vi "G#Object_ExternalCreateProcessDelegate.vi"(0 "delegate event out":refnum<user-event>, 1 "event queue":refnum<queue>, 5 "error in (no error)":errorcluster) -> (19 "error out":errorcluster)   [LabVIEW 2017, in "G#Object.lvclass"]
doc: "This is a delegate process that creates the object specified by the events."
uses:
  G#Object.lvclass
  utils/G#Object_Event.ctl
  utils/G#Object_EventType.ctl
  utils/G#Object_ObjectInfoType.ctl
  utils/G#Object_CreateMethod.ctl
  <vilib>/Utility/error.llb/Error Cluster From Error Code.vi
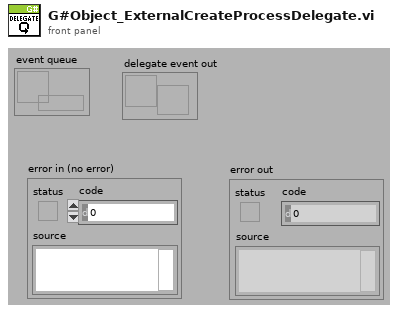
[diagram p1: front panel]
types:
  T1 = typedef "G#Object.lvclass/G#Object_EventType.ctl" = enum16{"Created new", "Looked up existing", "Deleted", "Forced delete", "Not deleted", "Garbage collected", "Cleared", "User", "Error", "External create object", "External create class attributes", "Created class attributes", "Run constructor", "Run constructor done", "Run open method", "Run open method done"}
  T2 = typedef "G#Object.lvclass/G#Object_ObjectInfoType.ctl" = cluster{"ObjectName":string, "ObjectID":u32, "Users":i32, "Counter":bool, "AttributeRefs":u32[], "FullClassName":string, "ClassName":string, "CreateMethod":T3, "GenericDestructorExists":bool, "Owner":string}
  T3 = typedef "G#Object.lvclass/G#Object_CreateMethod.ctl" = enum16{"Create", "Create or look up existing", "Look up existing"}
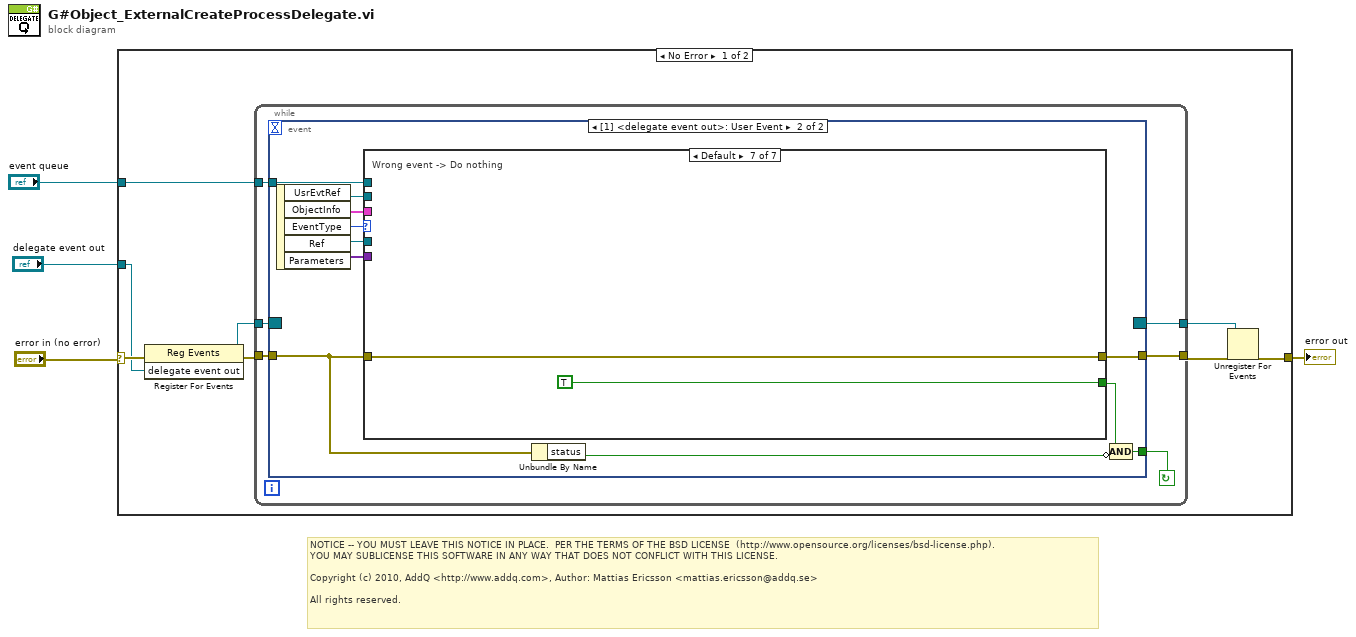
[diagram p0: block diagram]
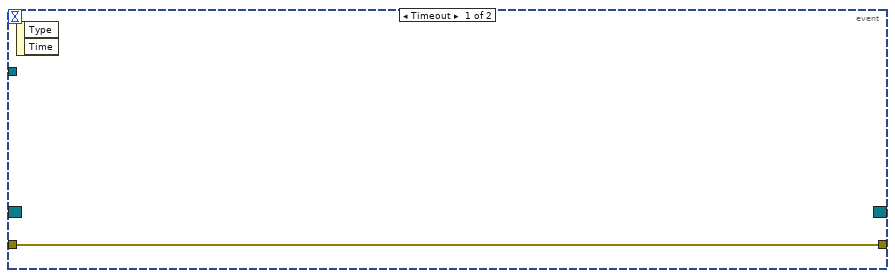
[diagram p2: hidden frame]
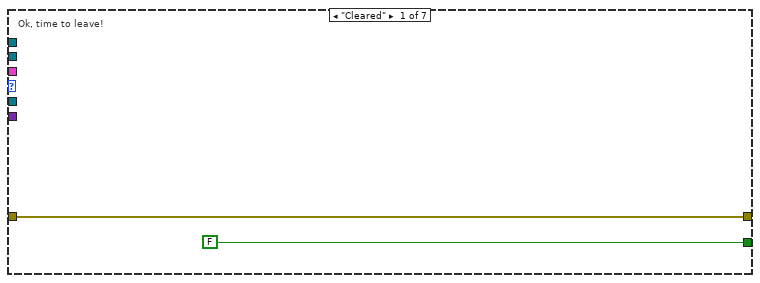
[diagram p3: hidden frame]
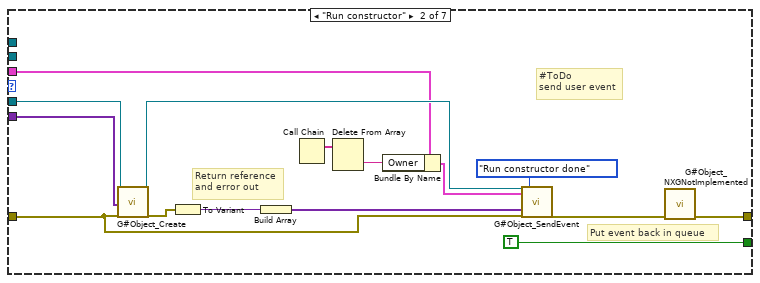
[diagram p4: hidden frame]
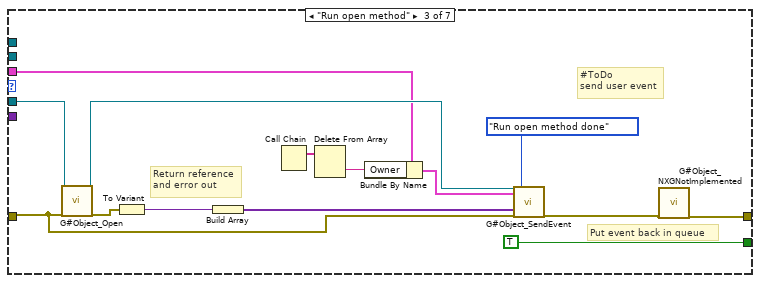
[diagram p5: hidden frame]
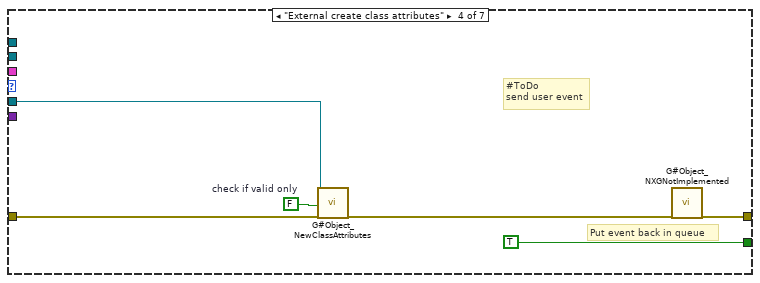
[diagram p6: hidden frame]
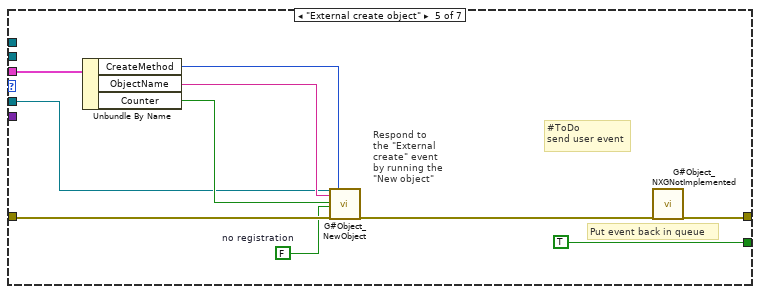
[diagram p7: hidden frame]
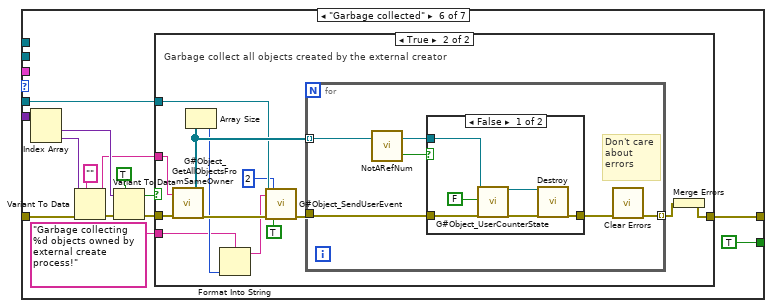
[diagram p8: hidden frame]
diagram:
  # "NOTICE -- YOU MUST LEAVE THIS NOTICE IN PLACE.  PER THE TERMS OF THE BSD LICENSE  (http://www.opensource.org/licenses/bsd-license.php).\nYOU MAY SUBLICENSE THIS SOFTWARE IN ANY WAY THAT DOES NOT CONFLICT WITH THIS LICENSE.\n\nCopyright (c) 2010, AddQ <http://www.addq.com>, Author: Mattias Ericsson <mattias.ericsson@addq.se>\n\nAll rights reserved."
  n1 = case shown="No Error" "error in (no error)" {
    selector: "error in (no error)" -> [w9 w121]
    tunnel: [w11 w121] -> w4
    tunnel: "event queue" -> [w12 _]
    tunnel: "delegate event out" -> [w8 _]
    frame No Error {
      n2 = register-events(error in=w9, w8) -> (reference out=w6:refnum<event-registration>, error out=w7:errorcluster)  [unwired: 1 in]
      n3 = while {
        tunnel: w7 -> [w18]
        tunnel: [w17] -> w10
        tunnel: w12 -> [w15]
        tunnel: w6 -> [w14]
        tunnel: [w13] -> w5
        stop <- w16 continue-if-true
        n4 = event shown="[1] <delegate event out>: User Event" {
          selector: w14 -> [_ _]
          dyn-events: [_ _] -> w13
          timeout: _ -> [_ _]
          tunnel: w18 -> [w19 w28]
          tunnel: [w19 w30] -> w17
          tunnel: [_ w25] -> w16
          tunnel: w15 -> [_ w22]
          event Timeout {
            n5 = event-data() -> ()  [unwired: 1 in, 2 out]
          }
          event User Event {
            n6 = event-data() -> ("UsrEvtRef"=w21:refnum<user-event>, "ObjectInfo"=w23:T2, "EventType"=w29:T1, "Ref"=w20:refnum<class "G#Object.lvclass">, "Parameters"=w24:variant[])  [unwired: 1 in]
            n7 = case shown="Default" w29 {
              tunnel: w28 -> [w32 w40 w54 w65 w73 w88 w119]
              tunnel: [w32 w33 w48 w62 w68 w90 w119] -> w30
              tunnel: [FALSE TRUE TRUE TRUE TRUE TRUE TRUE] -> w26
              tunnel: w24 -> [_ w35 _ _ _ w91 _]
              tunnel: w23 -> [_ w39 w51 _ w74 _ _]
              tunnel: w22 -> [_ _ _ _ _ _ _]
              tunnel: w21 -> [_ _ _ _ _ _ _]
              tunnel: w20 -> [_ w42 w56 w66 w71 w79 _]
              frame "Cleared" {
                # "Ok, time to leave!"
              }
              frame "Run constructor" {
                # "#ToDo\nsend user event"
                # "Put event back in queue"
                # "Return reference\nand error out"
                n8 = call-dynamic "G#Object_Create.vi"("reference in"=w42, "control values"=w35, "error in (no error)"=w40) -> ("reference out"=w41:refnum<class "G#Object.lvclass">, "error out"=w46:errorcluster)  [unwired: 15 in]
                n9 = To Variant(anything=w46) -> (Variant=w45:variant)
                n10 = Build Array(w45) -> (w43:variant[])
                n11 = Call Chain() -> (call chain=w37:string[])
                n12 = Delete From Array(array=w37) -> (deleted portion=w36:string)  [unwired: 2 in, 1 out]
                n13 = Bundle By Name(cluster=w39, "Owner"=w36) -> (w38:T2)
                n14 = call "G#Object_SendEvent.vi"("reference in"=w41, "object info extended"=w38, "parameters"=w43, "error in (no error)"=w40, "G# event type"=G#Object_EventType."Run constructor done") -> ("error out"=w34:errorcluster)  [unwired: 14 in]
                n15 = call "G#Object_NXGNotImplemented.vi"("error in"=w34) -> ("error out"=w33:errorcluster)  [unwired: 18 in]
              }
              frame "Run open method" {
                # "#ToDo\nsend user event"
                # "Put event back in queue"
                # "Return reference\nand error out"
                n16 = call-dynamic "G#Object_Open.vi"("reference in"=w56, "error in (no error)"=w54) -> ("reference out"=w55:refnum<class "G#Object.lvclass">, "error out"=w60:errorcluster)  [unwired: 16 in]
                n17 = To Variant(anything=w60) -> (Variant=w59:variant)
                n18 = Build Array(w59) -> (w57:variant[])
                n19 = Call Chain() -> (call chain=w53:string[])
                n20 = Delete From Array(array=w53) -> (deleted portion=w52:string)  [unwired: 2 in, 1 out]
                n21 = Bundle By Name(cluster=w51, "Owner"=w52) -> (w50:T2)
                n22 = call "G#Object_SendEvent.vi"("reference in"=w55, "object info extended"=w50, "parameters"=w57, "error in (no error)"=w54, "G# event type"=G#Object_EventType."Run open method done") -> ("error out"=w49:errorcluster)  [unwired: 14 in]
                n23 = call "G#Object_NXGNotImplemented.vi"("error in"=w49) -> ("error out"=w48:errorcluster)  [unwired: 18 in]
              }
              frame "External create class attributes" {
                w64 = FALSE  # check if valid only
                # "#ToDo\nsend user event"
                # "Put event back in queue"
                n24 = call "G#Object_NewClassAttributes.vi"("reference in"=w66, "check if valid only (F)"=w64, "error in (no error)"=w65) -> ("error out"=w63:errorcluster)  [unwired: 12 in, 4 out]
                n25 = call "G#Object_NXGNotImplemented.vi"("error in"=w63) -> ("error out"=w62:errorcluster)  [unwired: 18 in]
              }
              frame "External create object" {
                w70 = FALSE  # no registration
                # "#ToDo\nsend user event"
                # "Put event back in queue"
                # "Respond to\nthe \"External\ncreate\" event\nby running the\n\"New object\""
                n26 = Unbundle By Name(w74) -> ("CreateMethod"=w77:T3, "ObjectName"=w76:string, "Counter"=w75:bool)
                n27 = call "G#Object_NewObject.vi"("reference in"=w71, "object name (\"\")"=w76, "user counter (T)"=w75, "no registration (F)"=w70, "error in (no error)"=w73, "create method"=w77) -> ("error out"=w69:errorcluster)  [unwired: 11 in, 2 out]
                n28 = call "G#Object_NXGNotImplemented.vi"("error in"=w69) -> ("error out"=w68:errorcluster)  [unwired: 18 in]
              }
              frame "Garbage collected" {
                n29 = Index Array(array=w91) -> (element #1=w84:variant, element #2=w85:variant)  [unwired: 2 in]
                n30 = Variant To Data(error in=w88, type="", Variant=w85) -> (data=w80:string, error out=w87:errorcluster)
                n31 = Variant To Data(error in=w87, type=TRUE, Variant=w84) -> (data=w81:bool, error out=w86:errorcluster)
                n32 = case shown="True" w81 {
                  tunnel: [w92 w105] -> w90
                  tunnel: w86 -> [w92 w103]
                  tunnel: w80 -> [_ w102]
                  tunnel: w79 -> [_ w98]
                  tunnel: "Garbage collecting %d objects owned by external create process!" -> [_ w95]
                  frame False {
                  }
                  frame True {
                    # "Garbage collect all objects created by the external creator"
                    n33 = call "G#Object_GetAllObjectsFromSameOwner.vi"("full class name (\"\")"=w102, "error in (no error)"=w103) -> ("all refs"=w101:refnum<class "G#Object.lvclass">[], "error out"=w100:errorcluster)  [unwired: 14 in, 2 out]
                    n34 = Array Size(array=w101) -> (size(s)=w97:i32)
                    n35 = Format Into String(format string=w95, w97) -> (resulting string=w96:string)  [unwired: 2 in, 1 out]
                    n36 = call "G#Object_SendUserEvent.vi"("refererence in"=w98, "text"=w96, "error in (no error)"=w100, "call depth (1)"=2 ("call depth"), "send to Desktop Trace Execution? (F)"=TRUE ("send to Desktop Trace Execution")) -> ("error out"=w99:errorcluster)  [unwired: 13 in, 1 out]
                    n37 = for {
                      tunnel: w99 -> [w106]
                      tunnel: [w110] -> w104 mode=indexing
                      tunnel: w101 -> [w109] mode=indexing
                      # "Don't care\nabout\nerrors"
                      n38 = call-dynamic "NotARefNum.vi"("reference in"=w109) -> ("not a refnum?"=w108:bool, "reference out"=w107:refnum<class "G#Object.lvclass">)  [unwired: 1 in]
                      n39 = case shown="False" w108 {
                        tunnel: [w117 w118] -> w111
                        tunnel: w106 -> [w116 w118]
                        tunnel: w107 -> [w114 _]
                        frame False {
                          n40 = call "G#Object_UserCounterState.vi"("reference in"=w114, "user counter (F)"=FALSE, "error in (no error)"=w116) -> ("reference out"=w112:refnum<class "G#Object.lvclass">, "error out"=w115:errorcluster)  [unwired: 15 in]
                          n41 = call-dynamic "Destroy.vi"("reference in"=w112, "error in (no error)"=w115) -> ("error out"=w117:errorcluster)  [unwired: 16 in, 1 out]
                        }
                        frame True {
                        }
                      }
                      n42 = call <vilib>:"Clear Errors.vi"("error in (no error)"=w111) -> ("error out"=w110:errorcluster)  [unwired: 5 in, 1 out]
                    }
                    n43 = Merge Errors(w104) -> (w105:errorcluster)
                  }
                }
              }
              frame Default {
                # "Wrong event -> Do nothing"
              }
            }
            n44 = Unbundle By Name(w28) -> ("status"=w27:bool)
            n45 = Compound Arithmetic op=AND(w26, invert w27) -> (w25:bool)
          }
        }
      }
      n46 = Unregister For Events(event registration refnum=w5, error in=w10) -> (error out=w11:errorcluster)
    }
    frame Error {
    }
  }
  "error out" <- w4
